vi "Unregister Track.vi"(6 "Track ID":u64, 8 "error in":errorcluster) -> (0 "error out":errorcluster)   [LabVIEW 2023, in "VS Tracing API.lvlib"]
doc: "Closes and removes a previously registered custom track.\nCall this VI when tracing is complete and no further events will be recorded on the track.\n\n<b>Parameters</b>\n• <b>Track ID</b>: Identifier of the track to unregister.\n\n<b>Notes</b>\n• The Track ID must match a track previously created using <i>Register Track</i>.\n• Any events on the track should be completed before unregistering the track."
uses:
  VS Tracing API.lvlib
  libvs_perfetto.dll
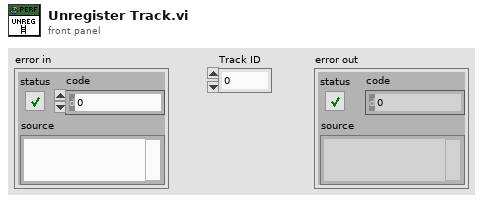
[diagram p1: front panel]
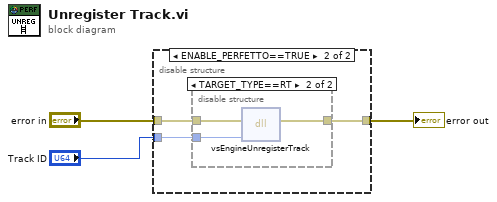
[diagram p0: block diagram]
diagram:
  n1 = disable-structure shown="ENABLE_PERFETTO==TRUE" {
    disable-tunnel: "error in" -> [w4 w6]
    disable-tunnel: [w4 w7] -> w2
    disable-tunnel: "Track ID" -> [_ w5]
    frame condition #0 (active) {
    }
    frame condition #1 {
      n2 = disable-structure shown="TARGET_TYPE==RT" {
        disable-tunnel: [w8 w11] -> w7
        disable-tunnel: w6 -> [w8 w10]
        disable-tunnel: w5 -> [_ w9]
        frame condition #0 (active) {
        }
        frame condition #1 {
          n3 = dll-call lib="libvs_perfetto.*" fn="vsEngineUnregisterTrack"(error in=w10, "trackId"=w9) -> (error out=w11:errorcluster)  [unwired: 4 in, 1 out]
        }
      }
    }
  }
  "error out" <- w2
